vi "SW-Microscoper.vi"(1 "Number of Scans to Average":i32=1 min=1 max=10000 step=1, 2 "Integration Time (ms)":i32=20 caption="Inter scan delay ms" min=10 step=10) -> ()   [LabVIEW 2012]
uses:
  Spectrometer/Events/SpectrometerEvents.ctl
  typedefs/Filenaming.ctl
  Spectrometer/SpectrometerSpectraWiz.llb/StellarNet Globals.vi
  variables/GlobalUI.vi
  <vilib>/Utility/file.llb/Write To Spreadsheet File (string).vi
  <vilib>/Utility/file.llb/Write To Spreadsheet File (DBL).vi
panel:
  in  "1000 ms":bool
  in  "20ms":bool
  in  "File Description":string
  out "Intensity":dbl
  out "Wavelength":dbl
  in  "Watts":bool=TRUE
  in  "Normalize":bool
  in  "Enable fit":bool
  in  "Reset Graph":bool
  out "FWHM":dbl=12.0
  out "Center (nm)":dbl=785.070003461609
  in  "Offset":dbl step=500.0
  in  "FWHM":dbl=12.0
  out "Background":sgl[][](array[numeric])
  in  "Continuous":bool
  out "Spectrometer data array sizes":i32[](array[numeric])=[2047]
  out "Spectrometer wavelengths":sgl[][](array[numeric])=[[337.41, 337.9242, 338.4383, 338.95227, 339.46616, 339.97992, 340.4936, 341.00717, 341.52063, 342.03397, 342.54724, 343.06036, 343.57343, 344.08633, 344.59918, 345.11188, 345.6245, 346.13702, 346.6494, 347.1617, 347.67392, 348.186, 348.698, 349.20987, 349.72165, 350.2333, 350.74487, 351.25632, 351.76767, 352.27893, 352.79007, 353.30112, 353.81204, 354.32285, 354.8336, 355.34418, 355.8547, 356.3651, 356.8754, 357.3856, 357.8957, 358.40567, 358.91553, 359.4253, 359.93497, 360.44452, 360.95398, 361.46335, 361.97256, 362.48172, 362.99075, 363.49966, 364.0085, 364.5172, 365.02582, 365.53433, 366.04272, 366.55103, 367.0592, 367.5673, 368.0753, 368.58316, 369.0909, 369.59857, 370.10614, 370.6136, 371.12094, 371.62817, 372.1353, 372.64233, 373.14926, 373.6561, 374.1628, 374.6694, 375.1759, 375.6823, 376.1886, 376.6948, 377.20087, 377.70685, 378.2127, 378.71848, 379.22415, 379.7297, 380.23514, 380.74048, 381.24573, 381.75085, 382.2559, 382.7608, 383.26562, 383.77036, 384.27493, 384.77945, 385.28384, 385.78815, 386.29233, 386.7964, 387.30035, 387.80423, 388.308, 388.81165, 389.31522, 389.81866, 390.322, 390.82523, 391.32837, 391.8314, 392.33432, 392.83713, 393.33984, 393.84244, 394.34494, 394.84732, 395.3496, 395.8518, 396.35388, 396.85583, 397.3577, 397.85947, 398.3611, 398.86267, 399.3641, 399.86545, 400.3667, 400.8678, 401.36884, 401.86975, 402.37057, 402.87128, 403.37186, 403.87238, 404.37274, 404.87305, 405.37323, 405.8733, 406.37326, 406.87314, 407.3729, 407.87253, 408.37207, 408.87152, 409.37085, 409.8701, 410.3692, 410.86823, 411.36716, 411.86597, 412.36465, 412.86325, 413.36176, 413.86014, 414.35843, 414.8566, 415.35468, 415.85263, 416.3505, 416.84824, 417.3459, 417.84344, 418.34088, 418.83823, 419.33545, 419.83255, 420.3296, 420.8265, 421.3233, 421.82, 422.3166, 422.81308, 423.30948, 423.80576, 424.3019, 424.798, 425.29395, 425.78983, 426.28555, 426.78122, 427.27676, 427.7722, 428.26752, 428.76276, 429.25787, 429.75287, 430.2478, 430.74258, 431.2373, 431.73187, 432.22638, 432.72076, 433.21503, 433.7092, 434.20328, 434.69724, 435.19107, 435.68484, 436.17847, 436.67203, 437.16544, 437.65878, 438.152, 438.6451, 439.13812, 439.63104, 440.12384, 440.61655, 441.10913, 441.6016, 442.094, 442.58627, 443.07843, 443.5705, 444.06244, 444.5543, 445.04605, 445.5377, 446.02924, 446.52066, 447.012, 447.5032, 447.99432, 448.48532, 448.97623, 449.46704, 449.95773, 450.4483, 450.93878, 451.42917, 451.91943, 452.4096, 452.89966, 453.38962, 453.8795, 454.36923, 454.85886, 455.3484, 455.83783, 456.32715, 456.81638, 457.30548, 457.7945, 458.2834, 458.7722, 459.26086, 459.74945, 460.23795, 460.72632, 461.21457, 461.70273, 462.1908, 462.67874, 463.1666, 463.65433, 464.14197, 464.62952, 465.11694, 465.60425, 466.09146, 466.57858, 467.06558, 467.5525, 468.03928, 468.52597, 469.01254, 469.49902, 469.98538, 470.47165, 470.95782, 471.44388, 471.92984, 472.41568, 472.9014, 473.38705, 473.87256, 474.358, 474.84332, 475.32852, 475.81363, 476.29865, 476.78354, 477.2683, 477.753, 478.23758, 478.72205, 479.20642, 479.6907, 480.17487, 480.6589, 481.14285, 481.62668, 482.11044, 482.59406, 483.07758, 483.561, 484.0443, 484.52753, 485.01065, 485.49362, 485.97653, 486.45932, 486.942, 487.4246, 487.90704, 488.3894, 488.87167, 489.35382, 489.83588, 490.31784, 490.79965, 491.2814, 491.76303, 492.24457, 492.72598, 493.20728, 493.68848, 494.1696, 494.65057, 495.13147, 495.61227, 496.09296, 496.57352, 497.054, 497.53436, 498.01462, 498.49475, 498.97482, 499.45474, 499.9346, 500.41434, 500.89395, 501.37347, 501.85287, 502.33218, 502.8114, 503.2905, 503.7695, 504.24838, 504.72717, 505.20584, 505.68442, 506.16287, 506.64124, 507.1195, 507.59766, 508.07568, 508.55362, 509.03146, 509.5092, 509.98682, 510.46432, 510.94174, 511.41907, 511.89627, 512.37335, 512.85034, 513.3272, 513.804, 514.2807, 514.75726, 515.2337, 515.7101, 516.18634, 516.6625, 517.13855, 517.61444, 518.0903, 518.56604, 519.0416, 519.51715, 519.99255, 520.4679, 520.94305, 521.41815, 521.8931, 522.36804, 522.84283, 523.3175, 523.79205, 524.26654, 524.74084, 525.21515, 525.6893, 526.1633, 526.63727, 527.1111, 527.5848, 528.0584, 528.5319, 529.0053, 529.47864, 529.95184, 530.4249, 530.8979, 531.3708, 531.84357, 532.3162, 532.7888, 533.2612, 533.7336, 534.2059, 534.678, 535.15, 535.62195, 536.0938, 536.5655, 537.0371, 537.50867, 537.98004, 538.45135, 538.92255, 539.3936, 539.8646, 540.3355, 540.8063, 541.2769, 541.7475, 542.21796, 542.6883, 543.15857, 543.62866, 544.0987, 544.56866, 545.03845, 545.5082, 545.9778, 546.4473, 546.9167, 547.386, 547.8552, 548.3243, 548.7933, 549.26215, 549.7309, 550.1996, 550.66815, 551.1366, 551.6049, 552.0732, 552.5413, 553.00934, 553.4773, 553.9451, 554.41284, 554.88043, 555.34796, 555.8153, 556.28265, 556.7498, 557.2169, 557.6839, 558.15076, 558.6175, 559.08417, 559.5507, 560.0172, 560.4835, 560.94977, 561.4159, 561.88196, 562.34784, 562.81366, 563.2794, 563.745, 564.2105, 564.6759, 565.1412, 565.6064, 566.0715, 566.53644, 567.0013, 567.46606, 567.9307, 568.39526, 568.85974, 569.3241, 569.7883, 570.25244, 570.7165, 571.1804, 571.6442, 572.1079, 572.57153, 573.03503, 573.4984, 573.96173, 574.42487, 574.888, 575.35095, 575.8138, 576.27655, 576.73926, 577.2018, 577.66425, 578.1266, 578.5888, 579.0509, 579.51294, 579.97485, 580.4367, 580.8984, 581.36, 581.8215, 582.2829, 582.7442, 583.2054, 583.66644, 584.1274, 584.58826, 585.049, 585.5097, 585.9702, 586.43066, 586.891, 587.35126, 587.81134, 588.27136, 588.7313, 589.1911, 589.6508, 590.1104, 590.56995, 591.0293, 591.4886, 591.94775, 592.40686, 592.8658, 593.32465, 593.78345, 594.24207, 594.7006, 595.15906, 595.61743, 596.0756, 596.53375, 596.99176, 597.4497, 597.9075, 598.3652, 598.8228, 599.2803, 599.7377, 600.19495, 600.65216, 601.1092, 601.56616, 602.023, 602.4798, 602.93646, 603.393, 603.8494, 604.3057, 604.76196, 605.2181, 605.67413, 606.13, 606.5858, 607.0415, 607.49713, 607.95264, 608.408, 608.8633, 609.3185, 609.7735, 610.22845, 610.68335, 611.1381, 611.5927, 612.0473, 612.5017, 612.95605, 613.4103, 613.8644, 614.3184, 614.77234, 615.22614, 615.6798, 616.1334, 616.5869, 617.0403, 617.4935, 617.9467, 618.3998, 618.8527, 619.3056, 619.75836, 620.211, 620.6635, 621.11597, 621.5683, 622.0205, 622.47266, 622.9246, 623.3765, 623.82837, 624.28, 624.7316, 625.1831, 625.6345, 626.08575, 626.5369, 626.988, 627.43896, 627.88983, 628.3406, 628.7912, 629.24176, 629.69214, 630.1425, 630.5927, 631.04285, 631.49286, 631.94275, 632.3925, 632.8422, 633.2918, 633.7413, 634.1907, 634.63995, 635.0891, 635.53815, 635.9871, 636.436, 636.8847, 637.3334, 637.78186, 638.2303, 638.67865, 639.12683, 639.57495, 640.02295, 640.4709, 640.91864, 641.36633, 641.81396, 642.2614, 642.7088, 643.15607, 643.6032, 644.0503, 644.49725, 644.9441, 645.3908, 645.83746, 646.284, 646.7304, 647.17676, 647.6229, 648.06903, 648.5151, 648.96094, 649.40674, 649.8524, 650.29803, 650.74347, 651.18884, 651.63416, 652.0793, 652.52435, 652.9693, 653.4141, 653.8589, 654.3035, 654.74805, 655.19244, 655.6368, 656.081, 656.5251, 656.9691, 657.413, 657.8568, 658.3005, 658.7441, 659.1875, 659.6309, 660.07416, 660.51733, 660.9604, 661.4033, 661.8461, 662.2889, 662.7315, 663.1741, 663.61646, 664.0588, 664.501, 664.9431, 665.3851, 665.82697, 666.2688, 666.71045, 667.15204, 667.5935, 668.03485, 668.47614, 668.9173, 669.35834, 669.79926, 670.2401, 670.68085, 671.12146, 671.562, 672.00244, 672.44275, 672.88293, 673.32306, 673.76306, 674.20294, 674.6427, 675.0824, 675.522, 675.9614, 676.4008, 676.84, 677.2792, 677.71826, 678.15717, 678.596, 679.0348, 679.4734, 679.9119, 680.35034, 680.78864, 681.2268, 681.6649, 682.1029, 682.54083, 682.9786, 683.41626, 683.8538, 684.2913, 684.7287, 685.16595, 685.6031, 686.0401, 686.47705, 686.9139, 687.35065, 687.78723, 688.22375, 688.66016, 689.0965, 689.53265, 689.96875, 690.4048, 690.84064, 691.2764, 691.7121, 692.1477, 692.5831, 693.0185, 693.45374, 693.8889, 694.3239, 694.75885, 695.1937, 695.6284, 696.06305, 696.49756, 696.932, 697.3663, 697.8005, 698.23456, 698.6686, 699.1024, 699.5362, 699.9699, 700.40344, 700.8369, 701.27026, 701.70355, 702.13666, 702.5697, 703.0026, 703.4355, 703.8682, 704.30084, 704.73334, 705.1657, 705.598, 706.0302, 706.46234, 706.8943, 707.3262, 707.75793, 708.18964, 708.6212, 709.0527, 709.484, 709.9152, 710.3464, 710.7774, 711.2084, 711.63916, 712.0699, 712.50055, 712.931, 713.36145, 713.79175, 714.2219, 714.65204, 715.082, 715.5119, 715.94165, 716.37134, 716.8009, 717.23035, 717.65967, 718.0889, 718.51807, 718.9471, 719.37604, 719.8049, 720.2336, 720.6622, 721.0907, 721.5191, 721.9474, 722.37555, 722.80365, 723.2316, 723.65955, 724.0873, 724.51495, 724.9425, 725.37, 725.7973, 726.22455, 726.6517, 727.07874, 727.5057, 727.9325, 728.3592, 728.78577, 729.2123, 729.6387, 730.065, 730.4912, 730.91724, 731.34326, 731.7691, 732.1949, 732.62054, 733.0461, 733.47156, 733.8969, 734.32214, 734.74725, 735.1723, 735.5972, 736.02203, 736.4468, 736.87134, 737.29584, 737.7203, 738.14453, 738.5687, 738.9928, 739.4168, 739.84064, 740.2644, 740.6881, 741.11163, 741.5351, 741.95844, 742.38165, 742.8048, 743.22784, 743.65076, 744.07355, 744.4963, 744.9189, 745.3414, 745.76373, 746.18604, 746.6082, 747.03033, 747.4523, 747.87415, 748.2959, 748.7176, 749.1391, 749.56055, 749.98193, 750.40314, 750.8243, 751.2453, 751.6662, 752.08704, 752.50775, 752.92834, 753.3488, 753.7692, 754.1895, 754.6097, 755.0298, 755.4497, 755.86957, 756.28937, 756.709, 757.12854, 757.548, 757.96735, 758.3866, 758.8057, 759.22473, 759.6436, 760.06244, 760.48114, 760.8997, 761.31824, 761.73663, 762.1549, 762.5731, 762.99115, 763.4091, 763.82697, 764.24475, 764.6624, 765.07996, 765.4974, 765.91473, 766.332, 766.7491, 767.1661, 767.583, 767.9998, 768.4165, 768.8331, 769.2496, 769.666, 770.0823, 770.4985, 770.9145, 771.3305, 771.74634, 772.1621, 772.57776, 772.9933, 773.4087, 773.82404, 774.23926, 774.6544, 775.0694, 775.4843, 775.8991, 776.31384, 776.72845, 777.14294, 777.5573, 777.97156, 778.38574, 778.7998, 779.2138, 779.6276, 780.0414, 780.455, 780.8686, 781.282, 781.6953, 782.1086, 782.52167, 782.9347, 783.3476, 783.7604, 784.1731, 784.5857, 784.99817, 785.4106, 785.8228, 786.235, 786.6471, 787.059, 787.4709, 787.8826, 788.29425, 788.7058, 789.11725, 789.52856, 789.9398, 790.3509, 790.7619, 791.17285, 791.5836, 791.9943, 792.4049, 792.81537, 793.22577, 793.63605, 794.0462, 794.4563, 794.8662, 795.27606, 795.68585, 796.09546, 796.505, 796.9144, 797.3237, 797.733, 798.1421, 798.5511, 798.96, 799.3688, 799.77747, 800.1861, 800.59454, 801.0029, 801.4112, 801.8194, 802.2274, 802.6354, 803.0432, 803.451, 803.8586, 804.2661, 804.6736, 805.0809, 805.4881, 805.8952, 806.30225, 806.7091, 807.1159, 807.5226, 807.9292, 808.3357, 808.74207, 809.1483, 809.5545, 809.9605, 810.36646, 810.77234, 811.17804, 811.5837, 811.98926, 812.39465, 812.8, 813.2052, 813.6103, 814.0153, 814.4202, 814.825, 815.2297, 815.6343, 816.03876, 816.4431, 816.84735, 817.2515, 817.6556, 818.0595, 818.4634, 818.8671, 819.27075, 819.67426, 820.0777, 820.481, 820.8842, 821.28735, 821.6903, 822.0932, 822.49603, 822.8987, 823.3013, 823.70374, 824.10614, 824.50836, 824.9105, 825.3126, 825.71454, 826.1164, 826.5181, 826.91974, 827.3213, 827.7227, 828.124, 828.5252, 828.92633, 829.32733, 829.7282, 830.12897, 830.52966, 830.93024, 831.33075, 831.7311, 832.13135, 832.5315, 832.9315, 833.3315, 833.7313, 834.13104, 834.5307, 834.93024, 835.32965, 835.72894, 836.1282, 836.5272, 836.9263, 837.32513, 837.72394, 838.1226, 838.5212, 838.9196, 839.318, 839.71625, 840.1144, 840.51245, 840.9104, 841.3082, 841.70593, 842.1036, 842.5011, 842.8985, 843.29584, 843.69305, 844.09015, 844.4871, 844.88403, 845.2808, 845.6775, 846.07404, 846.4705, 846.8669, 847.2631, 847.65924, 848.0553, 848.45123, 848.8471, 849.2428, 849.6384, 850.03394, 850.4294, 850.82465, 851.21985, 851.615, 852.00995, 852.40485, 852.7996, 853.1943, 853.58887, 853.98334, 854.3777, 854.7719, 855.1661, 855.5601, 855.95404, 856.3479, 856.74164, 857.13525, 857.52875, 857.9222, 858.3154, 858.7087, 859.10175, 859.49475, 859.88763, 860.2804, 860.6731, 861.0656, 861.45807, 861.85046, 862.2427, 862.6348, 863.02686, 863.4188, 863.81067, 864.2024, 864.594, 864.9855, 865.3769, 865.7682, 866.1594, 866.5505, 866.94147, 867.33234, 867.72314, 868.1138, 868.50433, 868.89484, 869.28516, 869.6754, 870.06555, 870.45557, 870.8455, 871.23535, 871.62506, 872.0147, 872.4042, 872.7936, 873.18286, 873.5721, 873.9612, 874.35016, 874.739, 875.1278, 875.5165, 875.905, 876.29346, 876.6818, 877.07007, 877.4582, 877.84625, 878.2342, 878.622, 879.0097, 879.39734, 879.78485, 880.17224, 880.5595, 880.9467, 881.3338, 881.72076, 882.10767, 882.49445, 882.8811, 883.26764, 883.6541, 884.04047, 884.4267, 884.8128, 885.19885, 885.5848, 885.9706, 886.3563, 886.74194, 887.12744, 887.5128, 887.89813, 888.2833, 888.6684, 889.05334, 889.43823, 889.823, 890.20764, 890.5922, 890.9767, 891.361, 891.74524, 892.1294, 892.5134, 892.89734, 893.2812, 893.66486, 894.04846, 894.432, 894.81537, 895.19867, 895.58185, 895.9649, 896.3479, 896.7308, 897.1135, 897.4962, 897.8787, 898.26117, 898.64355, 899.02576, 899.4079, 899.7899, 900.1719, 900.55365, 900.93536, 901.31696, 901.6985, 902.0799, 902.4612, 902.84235, 903.22345, 903.6044, 903.9852, 904.366, 904.7467, 905.1272, 905.5077, 905.888, 906.26825, 906.6484, 907.0284, 907.4083, 907.78815, 908.16785, 908.5474, 908.92694, 909.30634, 909.6856, 910.06476, 910.44385, 910.8228, 911.2017, 911.58044, 911.9591, 912.33765, 912.71606, 913.0944, 913.47266, 913.85077, 914.2288, 914.60675, 914.98456, 915.36224, 915.7398, 916.1173, 916.4947, 916.872, 917.2492, 917.6262, 918.00323, 918.38007, 918.75684, 919.1335, 919.51, 919.8865, 920.2628, 920.63904, 921.01514, 921.3912, 921.7671, 922.1429, 922.5186, 922.89417, 923.26965, 923.6451, 924.0203, 924.3955, 924.77057, 925.14557, 925.5204, 925.89514, 926.26984, 926.64435, 927.0188, 927.3931, 927.76733, 928.1415, 928.5155, 928.8894, 929.2632, 929.6369, 930.0105, 930.384, 930.7574, 931.1306, 931.5038, 931.8769, 932.2498, 932.6227, 932.9954, 933.3681, 933.74066, 934.11304, 934.4854, 934.8576, 935.22974, 935.60175, 935.97363, 936.34546, 936.71716, 937.08875, 937.4602, 937.8316, 938.2029, 938.57404, 938.9451, 939.3161, 939.68695, 940.0577, 940.42834, 940.7989, 941.1693, 941.5396, 941.90985, 942.27997, 942.64996, 943.0199, 943.38965, 943.75934, 944.12897, 944.4984, 944.8678, 945.23706, 945.60626, 945.97534, 946.3443, 946.71313, 947.08185, 947.4505, 947.81903, 948.18744, 948.5558, 948.924, 949.2921, 949.66016, 950.028, 950.3958, 950.76355, 951.1311, 951.4986, 951.86597, 952.2332, 952.6004, 952.96747, 953.3344, 953.70123, 954.068, 954.43463, 954.80115, 955.1676, 955.53394, 955.90015, 956.26624, 956.63226, 956.99817, 957.36395, 957.7296, 958.0952, 958.4607, 958.82605, 959.19135, 959.5565, 959.9216, 960.2865, 960.65137, 961.0161, 961.38074, 961.74524, 962.1097, 962.474, 962.8382, 963.20233, 963.56635, 963.93024, 964.294, 964.6577, 965.02124, 965.38477, 965.7481, 966.1114, 966.47455, 966.8376, 967.20056, 967.56335, 967.92615, 968.28876, 968.6513, 969.0137, 969.37604, 969.7382, 970.10034, 970.46234, 970.8242, 971.18604, 971.5477, 971.9093, 972.27075, 972.63214, 972.9934, 973.35455, 973.7156, 974.07654, 974.4374, 974.7981, 975.15875, 975.5193, 975.8797, 976.24, 976.6002, 976.9603, 977.3203, 977.6802, 978.04, 978.39966, 978.7592, 979.1187, 979.4781, 979.83734, 980.1965, 980.55554, 980.9145, 981.2733, 981.632, 981.99066, 982.3492, 982.7076, 983.0659, 983.42413, 983.7822, 984.1402, 984.4981, 984.8559, 985.21356, 985.57117, 985.9286, 986.28595, 986.64325, 987.00037, 987.3574, 987.71436, 988.0712, 988.4279, 988.78455, 989.14105, 989.4975, 989.8538, 990.21, 990.5661, 990.9221, 991.27795, 991.6337, 991.98944, 992.34503, 992.70044, 993.05585, 993.4111, 993.76624, 994.1213, 994.4762, 994.83105, 995.1858, 995.5404, 995.8949, 996.2493, 996.60364, 996.9578, 997.3119, 997.6659, 998.0198, 998.3736, 998.72723, 999.0808, 999.43427, 999.78766, 1000.14087, 1000.494, 1000.84705, 1001.2, 1001.55286, 1001.9056, 1002.2582, 1002.6107, 1002.9631, 1003.3154, 1003.6676, 1004.0197, 1004.3717, 1004.7236, 1005.0753, 1005.427, 1005.77856, 1006.13, 1006.4814, 1006.83264, 1007.1838, 1007.5348, 1007.88574, 1008.2366, 1008.5873, 1008.9379, 1009.28845, 1009.63885, 1009.98914, 1010.33936, 1010.6894, 1011.0394, 1011.3893, 1011.7391, 1012.08875, 1012.4383, 1012.7877, 1013.1371, 1013.4863, 1013.83545, 1014.1845, 1014.53345, 1014.88226, 1015.231, 1015.5796, 1015.9281, 1016.2765, 1016.6248, 1016.973, 1017.3211, 1017.66907, 1018.01697, 1018.36475, 1018.7124, 1019.05994, 1019.4074, 1019.75476, 1020.102, 1020.44916, 1020.79614, 1021.14307, 1021.4899, 1021.8366, 1022.1832, 1022.5297, 1022.87616, 1023.2225, 1023.5686, 1023.91473, 1024.2607, 1024.6066, 1024.9524, 1025.298, 1025.6436, 1025.989, 1026.3344, 1026.6796, 1027.0248, 1027.3698, 1027.7147, 1028.0594, 1028.4042, 1028.7488, 1029.0934, 1029.4377, 1029.782, 1030.1262, 1030.4703, 1030.8142, 1031.1581, 1031.502, 1031.8456, 1032.1891, 1032.5326, 1032.8759, 1033.2191, 1033.5623, 1033.9053, 1034.2483, 1034.5911, 1034.9337, 1035.2764, 1035.6189, 1035.9613, 1036.3036, 1036.6458, 1036.9878, 1037.3298, 1037.6716, 1038.0134, 1038.3551, 1038.6967, 1039.0381, 1039.3794, 1039.7207, 1040.0618, 1040.4028, 1040.7438, 1041.0846, 1041.4253, 1041.7659, 1042.1063, 1042.4468, 1042.787, 1043.1272, 1043.4673, 1043.8073, 1044.1471, 1044.4869, 1044.8265, 1045.1661, 1045.5055, 1045.8448, 1046.1841, 1046.5232, 1046.8623, 1047.2012, 1047.54, 1047.8787, 1048.2173, 1048.5558, 1048.8942, 1049.2324, 1049.5707, 1049.9087, 1050.2467, 1050.5846, 1050.9224, 1051.26, 1051.5975, 1051.9349, 1052.2723, 1052.6095, 1052.9467, 1053.2837, 1053.6206, 1053.9574, 1054.2941, 1054.6307, 1054.9672, 1055.3036, 1055.6399, 1055.9761, 1056.3121, 1056.6481, 1056.9839, 1057.3197, 1057.6553, 1057.9908, 1058.3263, 1058.6616, 1058.9968, 1059.332, 1059.667, 1060.002, 1060.3368, 1060.6714, 1061.006, 1061.3406, 1061.6749, 1062.0092, 1062.3434, 1062.6775, 1063.0114, 1063.3452, 1063.679, 1064.0127, 1064.3462, 1064.6797, 1065.013, 1065.3462, 1065.6793, 1066.0123, 1066.3452, 1066.678, 1067.0107, 1067.3434, 1067.6758, 1068.0082, 1068.3405, 1068.6726, 1069.0048, 1069.3367, 1069.6686, 1070.0002, 1070.3319, 1070.6635, 1070.9949, 1071.3262, 1071.6575, 1071.9885, 1072.3196, 1072.6505, 1072.9813, 1073.312, 1073.6426, 1073.973, 1074.3035, 1074.6337, 1074.9639, 1075.294, 1075.6239, 1075.9537, 1076.2834, 1076.6132, 1076.9426, 1077.2721, 1077.6014, 1077.9307, 1078.2598, 1078.5887, 1078.9177, 1079.2465, 1079.5752, 1079.9038, 1080.2323, 1080.5607, 1080.8889, 1081.217, 1081.5452, 1081.873, 1082.2009, 1082.5287, 1082.8563, 1083.1838, 1083.5112, 1083.8386, 1084.1658, 1084.4929, 1084.82, 1085.1469, 1085.4736, 1085.8003, 1086.127, 1086.4534, 1086.7798, 1087.1061, 1087.4323, 1087.7583, 1088.0842, 1088.41, 1088.7358, 1089.0614, 1089.387, 1089.7124, 1090.0377, 1090.3629, 1090.688, 1091.0131, 1091.3379, 1091.6627, 1091.9874, 1092.312, 1092.6365, 1092.9608, 1093.2852, 1093.6093, 1093.9333, 1094.2573, 1094.5812, 1094.9049, 1095.2285, 1095.552, 1095.8755, 1096.1987, 1096.522, 1096.8451, 1097.1681, 1097.491, 1097.8137, 1098.1365, 1098.459, 1098.7815, 1099.1039, 1099.4261, 1099.7483, 1100.0703, 1100.3923, 1100.7141, 1101.0359, 1101.3575, 1101.6791, 1102.0005, 1102.3218, 1102.643, 1102.9641, 1103.2852, 1103.606, 1103.9268, 1104.2474, 1104.568, 1104.8885, 1105.2089, 1105.5292, 1105.8492, 1106.1693, 1106.4893, 1106.8091, 1107.1289, 1107.4485, 1107.7681, 1108.0874, 1108.4067, 1108.726, 1109.045, 1109.364, 1109.683, 1110.0017, 1110.3204, 1110.639, 1110.9574, 1111.2759, 1111.5941, 1111.9122, 1112.2302, 1112.5482, 1112.8661, 1113.1838, 1113.5015, 1113.819, 1114.1364, 1114.4536, 1114.7709, 1115.088, 1115.4049, 1115.7218, 1116.0386, 1116.3553, 1116.6719, 1116.9884, 1117.3047, 1117.621, 1117.9371, 1118.2532, 1118.5691, 1118.8849, 1119.2007, 1119.5162, 1119.8318, 1120.1472, 1120.4625, 1120.7777, 1121.0928, 1121.4078, 1121.7227, 1122.0375, 1122.3522, 1122.6667, 1122.9812, 1123.2955, 1123.6099, 1123.924, 1124.238, 1124.5519, 1124.8657, 1125.1794, 1125.4932, 1125.8066, 1126.12, 1126.4333, 1126.7466, 1127.0597, 1127.3727, 1127.6855, 1127.9983, 1128.3109, 1128.6235, 1128.936, 1129.2483, 1129.5605, 1129.8728, 1130.1848, 1130.4967, 1130.8086, 1131.1202, 1131.4319, 1131.7434, 1132.0548, 1132.3661, 1132.6774, 1132.9884, 1133.2994, 1133.6102, 1133.921, 1134.2317, 1134.5422, 1134.8528, 1135.1631, 1135.4734, 1135.7834, 1136.0935, 1136.4034, 1136.7133, 1137.023, 1137.3326, 1137.6421, 1137.9515, 1138.2609, 1138.5701, 1138.8792, 1139.1881, 1139.497, 1139.8058, 1140.1144, 1140.423, 1140.7314, 1141.0398, 1141.348, 1141.6561, 1141.9642, 1142.2721, 1142.58, 1142.8877, 1143.1953, 1143.5028, 1143.8102, 1144.1176, 1144.4247, 1144.7318, 1145.0388, 1145.3456, 1145.6525, 1145.9591, 1146.2656, 1146.5721, 1146.8784, 1147.1847, 1147.4908, 1147.7969, 1148.1028, 1148.4086, 1148.7144, 1149.0199, 1149.3254, 1149.6309, 1149.9362, 1150.2413, 1150.5464, 1150.8513, 1151.1562, 1151.461, 1151.7656, 1152.0702, 1152.3746, 1152.6791, 1152.9833, 1153.2874, 1153.5914, 1153.8954, 1154.1992, 1154.5029, 1154.8065, 1155.11, 1155.4135, 1155.7167, 1156.0199, 1156.323, 1156.626, 1156.9288, 1157.2316, 1157.5342, 1157.8368, 1158.1393, 1158.4415, 1158.7438, 1159.0459, 1159.348, 1159.6499, 1159.9517, 1160.2534, 1160.555, 1160.8566, 1161.158, 1161.4592, 1161.7604, 1162.0615, 1162.3624, 1162.6633, 1162.9641, 1163.2648, 1163.5653, 1163.8657, 1164.166, 1164.4663, 1164.7665, 1165.0664, 1165.3663, 1165.6661, 1165.966, 1166.2655, 1166.565, 1166.8644, 1167.1637, 1167.4629, 1167.762, 1168.0609, 1168.3597, 1168.6586, 1168.9572]]
  out "time elapsed prev scan (ms)":u32=270
  in  "Acquire Background":bool
  in  "Array":bool[](array[boolean])=[TRUE, TRUE, TRUE]
  out "Save paths":path[](array[path])=[path "C:/Users/Trent/Documents/Jeremy/2016-09-27/FW800 with Polarizer-100mW-417mW-0mV-0mV-0mV-4xch1_s_00.csv", path "C:/Users/Trent/Documents/Jeremy/2016-09-27/FW800 with Polarizer-100mW-417mW-0mV-0mV-0mV-4xch2_s_00.csv", path "C:/Users/Trent/Documents/Jeremy/2016-09-27/FW800 with Polarizer-100mW-417mW-0mV-0mV-0mV-4xch3_s_00.csv"]
  out "Numeric":i32=623
  in  "Init Trigger":bool
  in  "Autosave":bool
  in  "Acquire Trigger":bool
  in  "STOP":bool
  out "Spectral history":cluster{sgl, "lamda":sgl}[](graph)=[{0.12466025, "lamda"=796.9144}, {0.0966606, "lamda"=681.83813}, {0.06927186, "lamda"=985.23456}]
  out "Spectrum":T1(graph)
  # "BlackComet"
  # "BlueWave"
  # "DwarfStar"
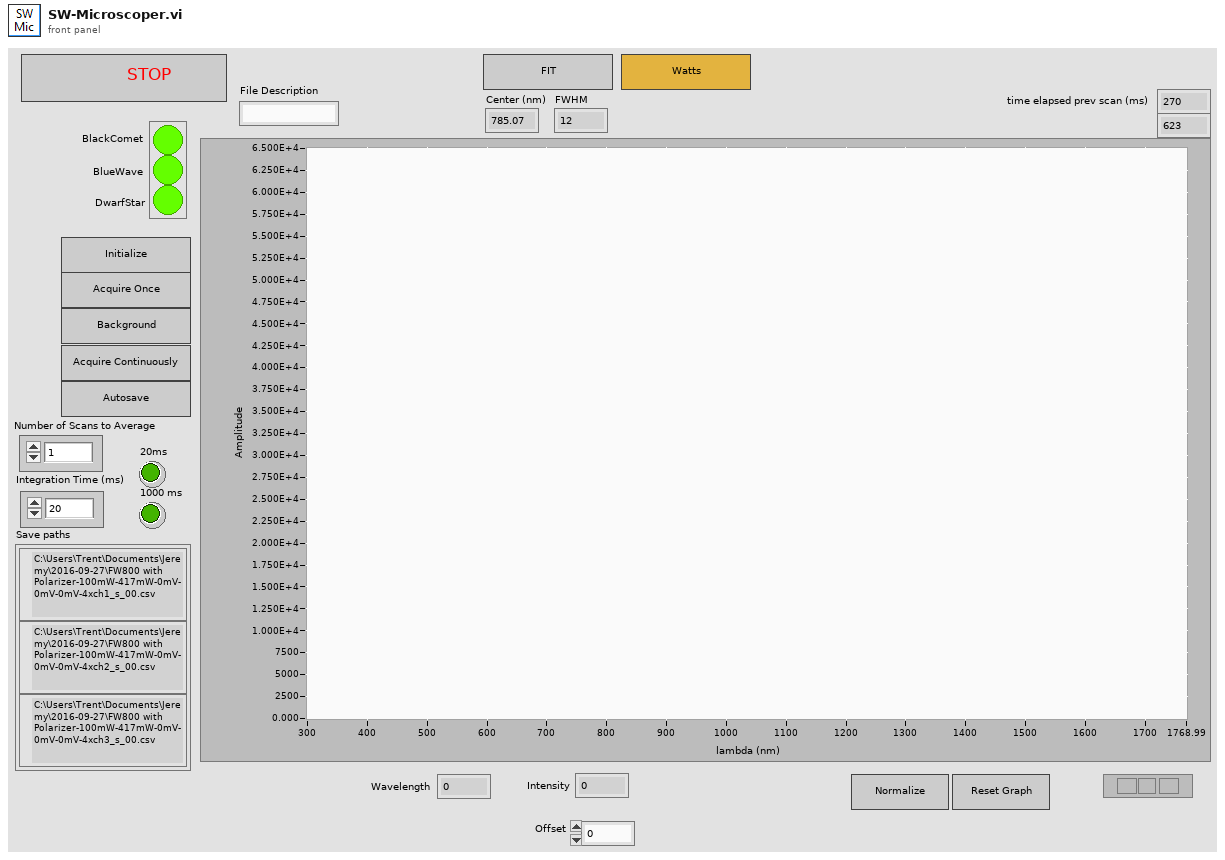
[diagram p1: front panel]
types:
  T1 = cluster{"Spectrometer wavelengths":sgl[], "buffer out":sgl[]}[]
  T2 = typedef "SpectrometerEvents.ctl" = enum16{"TimeOut", "Init Programmatically", "Init Button", "Init Background", "Acquire Background", "Acquire"}
  T3 = typedef "Filenaming.ctl" = enum16{"Image", "Just Description"}
  T4 = cluster{"Integration Time (msec)":i32, "Xtrate":i32, "Averaging":i32, "Smoothing":i32, "C1":dbl, "C2":dbl, "C3":dbl, "C4":dbl, "Digitizer Bits":enum8{"12", "14", "16"}}[]
  T5 = cluster{"Spectrometer wavelengths (filtered)":sgl[], "Normalized":dbl[]}
  T6 = cluster{"Spectrometer wavelengths (filtered)":sgl[], "Best Gaussian Fit":dbl[]}[]
  T7 = cluster{"Spectrometer wavelengths (filtered)":sgl[], "Normalized":sgl[]}
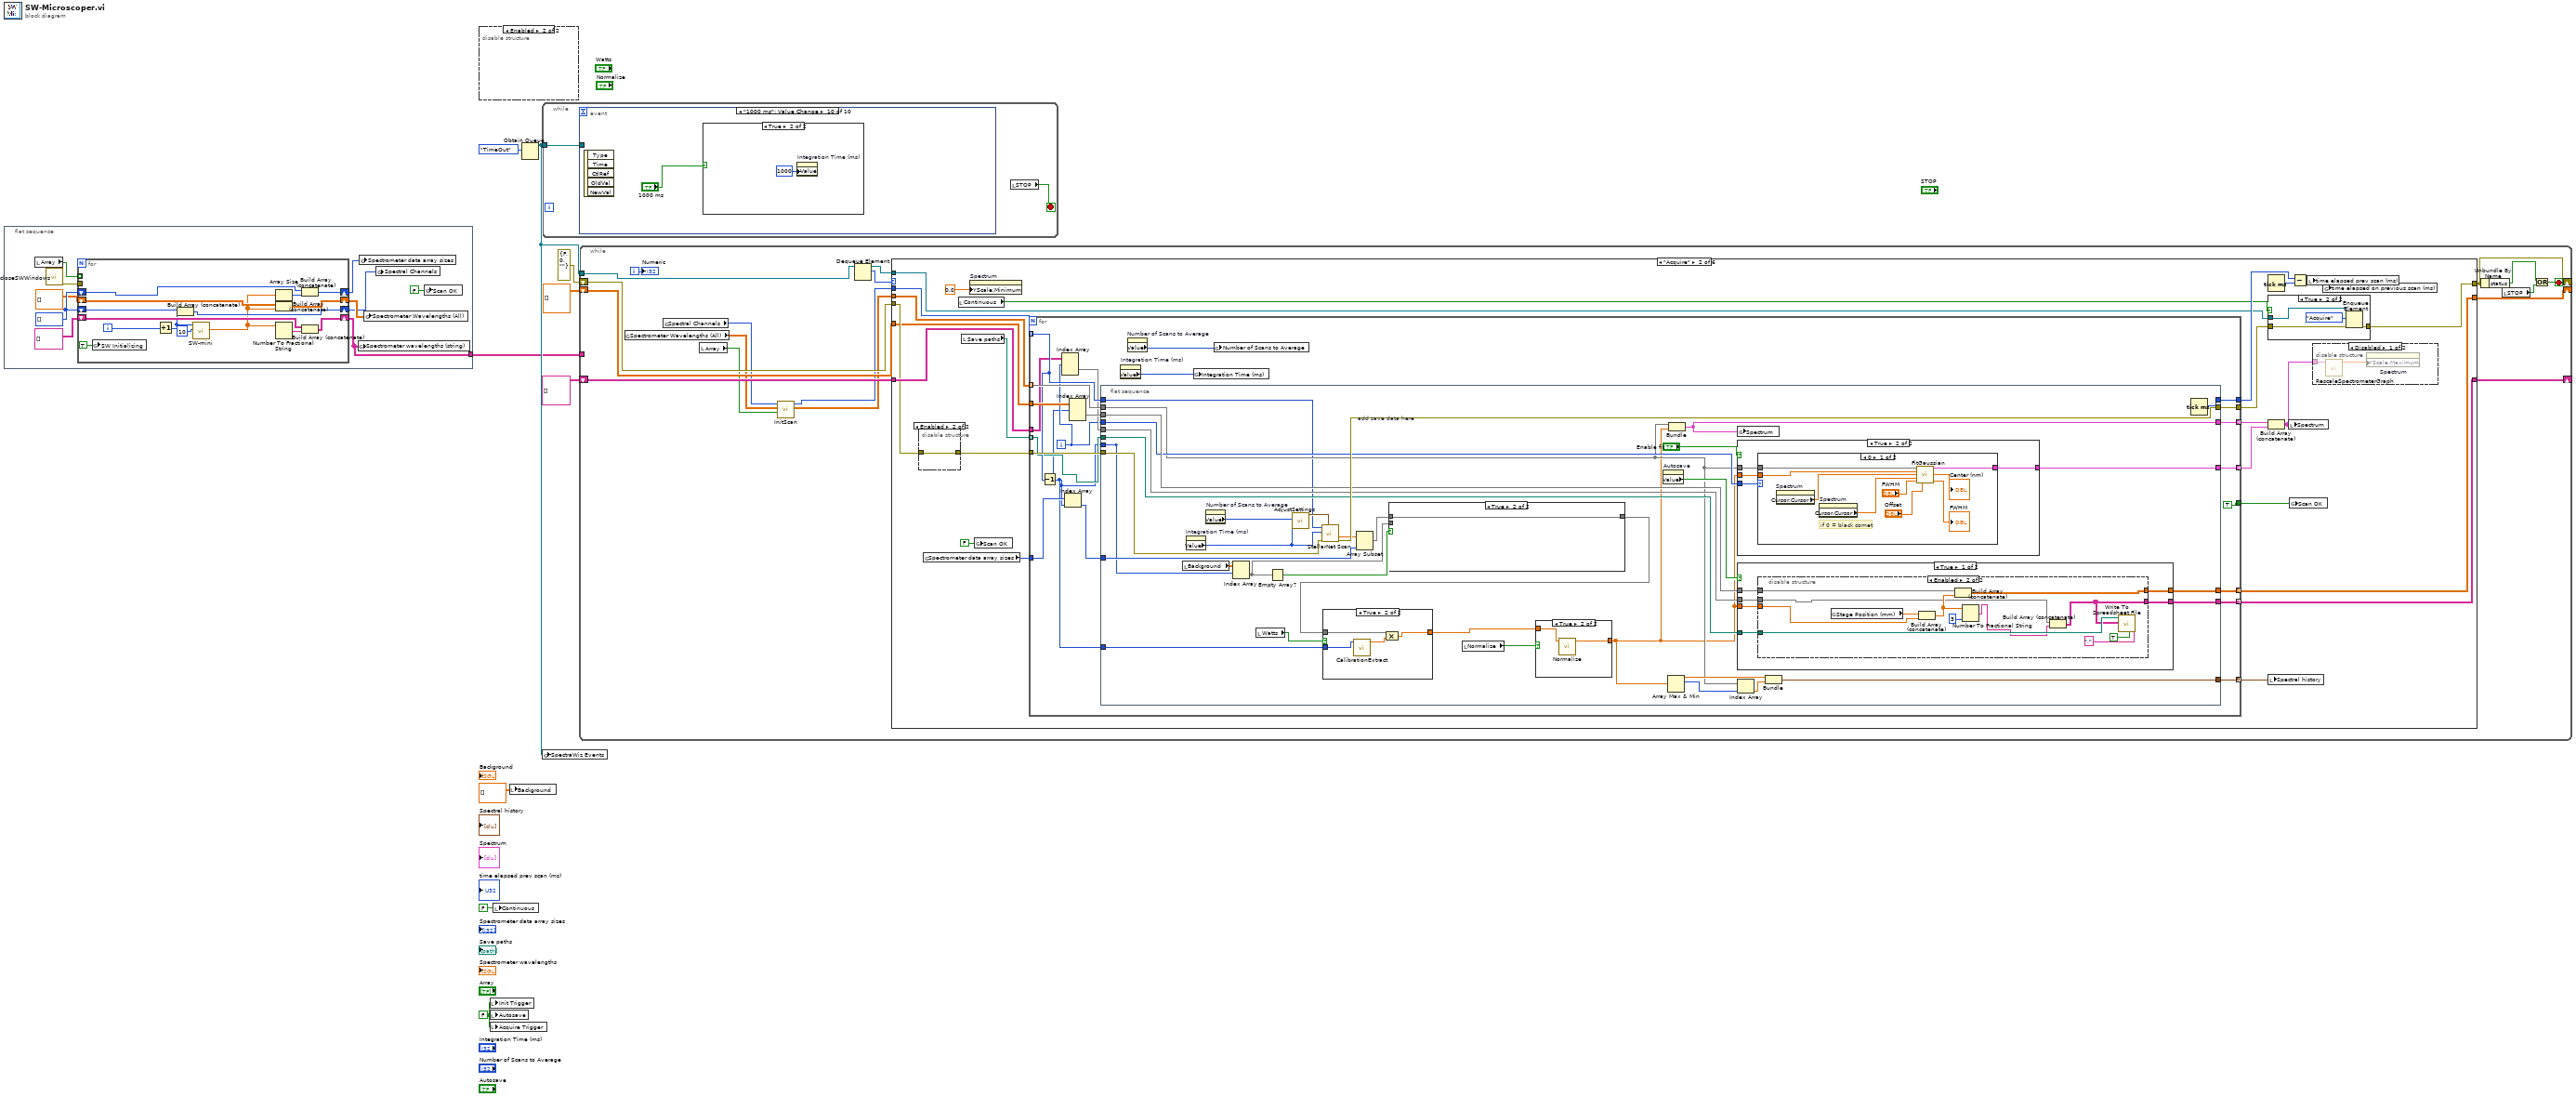
[diagram p0: block diagram]
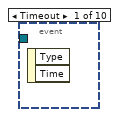
[diagram p2: hidden frame]
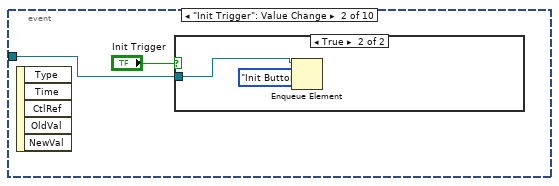
[diagram p3: hidden frame]
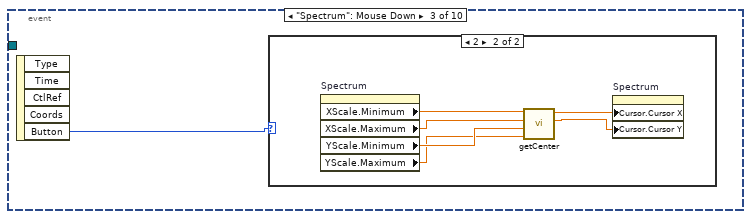
[diagram p5: hidden frame]
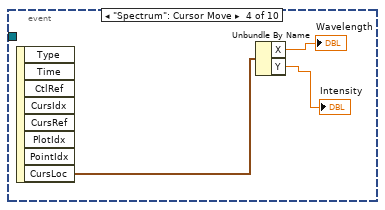
[diagram p7: hidden frame]
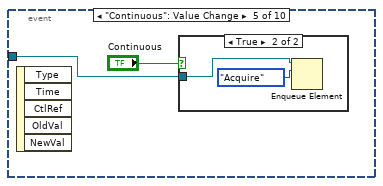
[diagram p8: hidden frame]
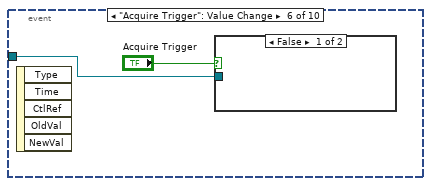
[diagram p10: hidden frame]
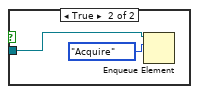
[diagram p11: hidden frame]
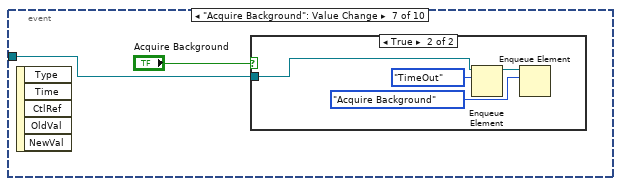
[diagram p12: hidden frame]
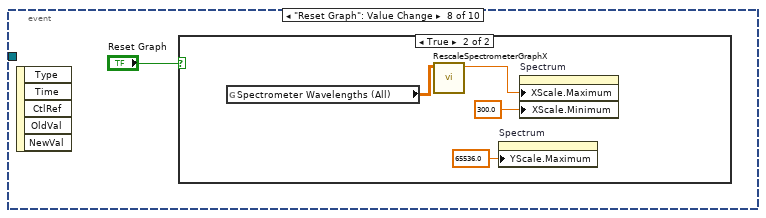
[diagram p14: hidden frame]
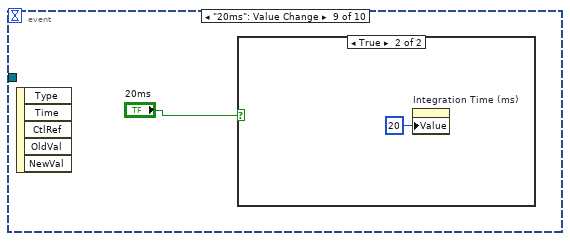
[diagram p16: hidden frame]
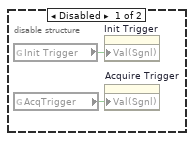
[diagram p19: hidden frame]
diagram:
  w2 = FALSE ("Init Trigger")
  n1 = flat-sequence {
    tunnel: [w11] -> w1
    frame #0 {
      w19 = i32[] []
      n2 = local read "Array"() -> (w17:bool[])
      n3 = call "closeSWWindows.vi"() -> ("error out"=w15:errorcluster)  [unwired: 11 in]
      n4 = for {
        tunnel: w17 -> [_] mode=indexing
        shift-right: [w33] -> w13
        shift-left: w19 -> [w32]
        tunnel: w15 -> [_]
        shift-right: [w30] -> w11
        shift-left: string[][] [] -> [w31]
        shift-right: [w28] -> w14
        shift-left: dbl[][] [] -> [w29]
        shift-right: [w27] -> w12
        shift-left: w19 -> [w26]
        i -> [w34]
        n5 = global write "GlobalUI.vi" "SW Initializing"(TRUE ("SW Initializing")) -> ()
        n6 = Increment(x=w34) -> (x+1=w25:i32)
        n7 = Build Array (concatenate)(w32, w25) -> (w33:i32[])
        n8 = call "SW-mini.vi"("Integration Time (ms)"=10, "Spectral Channel"=w25) -> ("Spectrometer wavelengths"=w22:sgl[])  [unwired: 6 in, 3 out]
        n9 = Array Size(array=w22) -> (size(s)=w21:i32)
        n10 = Build Array (concatenate)(w29, w22) -> (w28:dbl[][])
        n11 = Number To Fractional String(number=w22) -> (F-format string=w23:string[])  [unwired: 3 in]
        n12 = Build Array (concatenate)(w26, w21) -> (w27:i32[])
        n13 = Build Array (concatenate)(w31, w23) -> (w30:string[][])
      }
      n14 = global write "StellarNet Globals.vi" "Spectrometer wavelengths (string)"(w11) -> ()
      n15 = global write "StellarNet Globals.vi" "Spectrometer data array sizes"(w12) -> ()
      n16 = global write "StellarNet Globals.vi" "Spectrometer Wavelengths (All)"(w14) -> ()
      n17 = global write "StellarNet Globals.vi" "Spectral Channels"(w13) -> ()
      n18 = global write "StellarNet Globals.vi" "Scan OK"(FALSE ("Scan OK")) -> ()
    }
  }
  n19 = disable-structure shown="Enabled" {
    frame Disabled {
      n20 = global read "StellarNet Globals.vi" "Init Trigger"() -> (w36:bool)
      n21 = global read "StellarNet Globals.vi" "AcqTrigger"() -> (w35:bool)
      n22 = property on="Init Trigger" class="Bool (strict)"("Val(Sgnl)"=w36) -> ()  [unwired: 2 in, 2 out]
      n23 = property on="Acquire Trigger" class="Bool (strict)"("Val(Sgnl)"=w35) -> ()  [unwired: 2 in, 2 out]
    }
    frame Enabled {
    }
  }
  n24 = local write "Init Trigger"(w2) -> ()
  n25 = local write "Autosave"(w2) -> ()
  n26 = local write "Acquire Trigger"(w2) -> ()
  n27 = local write "Continuous"(FALSE ("Continuous")) -> ()
  n28 = local write "Background"(dbl[][] []) -> ()
  n29 = Obtain Queue(element data type=SpectrometerEvents."TimeOut" ("element")) -> (queue out=w5:refnum<queue>)  [unwired: 4 in, 2 out]
  n30 = while {
    tunnel: w5 -> [w38]
    stop <- w37 stop-if-true
    n31 = event shown="[9] \"1000 ms\": Value Change" {
      selector: _ -> [_ _ _ _ _ _ _ _ _ _]
      dyn-events: _ -> [_ _ _ _ _ _ _ _ _ _]
      timeout: _ -> [_ _ _ _ _ _ _ _ _ _]
      tunnel: w38 -> [_ w39 _ _ w54 w58 w62 _ _ _]
      event Timeout {
        n32 = event-data() -> ()  [unwired: 1 in, 2 out]
      }
      event "Init Trigger": Value Change {
        n33 = event-data() -> ()  [unwired: 1 in, 5 out]
        n34 = case shown="True" "Init Trigger" {
          tunnel: w39 -> [_ w42]
          frame False {
          }
          frame True {
            n35 = Enqueue Element(queue=w42, element=SpectrometerEvents."Init Button") -> ()  [unwired: 2 in, 3 out]
          }
        }
      }
      event "Spectrum": Mouse Down {
        n36 = event-data() -> ("Button"=w43:u16)  [unwired: 1 in, 4 out]
        n37 = case shown="2" w43 {
          frame 0, Default {
          }
          frame 2 {
            n38 = property on="Spectrum" class="XYGraph (strict)"() -> ("XScale.Minimum"=w49:dbl, "XScale.Maximum"=w48:dbl, "YScale.Minimum"=w47:dbl, "YScale.Maximum"=w46:dbl)  [unwired: 2 in, 2 out]
            n39 = call "getCenter.vi"("ymax"=w46, "ymin"=w47, "xmax"=w48, "xmin"=w49) -> ("y"=w44:dbl, "x"=w45:dbl)  [unwired: 6 in]
            n40 = property on="Spectrum" class="XYGraph (strict)"("Cursor.Cursor X"=w45, "Cursor.Cursor Y"=w44) -> ()  [unwired: 2 in, 2 out]
          }
        }
      }
      event "Spectrum": Cursor Move {
        n41 = event-data() -> ("CursLoc"=w52:cluster{"X":dbl, "Y":dbl})  [unwired: 1 in, 7 out]
        n42 = Unbundle By Name(w52) -> ("X"=→"Wavelength":dbl, "Y"=→"Intensity":dbl)
      }
      event "Continuous": Value Change {
        n43 = event-data() -> ()  [unwired: 1 in, 5 out]
        n44 = case shown="True" "Continuous" {
          tunnel: w54 -> [_ w56]
          frame False {
          }
          frame True {
            n45 = Enqueue Element(queue=w56, element=SpectrometerEvents."Acquire") -> ()  [unwired: 2 in, 3 out]
          }
        }
      }
      event "Acquire Trigger": Value Change {
        n46 = event-data() -> ()  [unwired: 1 in, 5 out]
        n47 = case shown="False" "Acquire Trigger" {
          tunnel: w58 -> [_ w60]
          frame False {
          }
          frame True {
            n48 = Enqueue Element(queue=w60, element=SpectrometerEvents."Acquire") -> ()  [unwired: 2 in, 3 out]
          }
        }
      }
      event "Acquire Background": Value Change {
        n49 = event-data() -> ()  [unwired: 1 in, 5 out]
        n50 = case shown="True" "Acquire Background" {
          tunnel: w62 -> [_ w66]
          frame False {
          }
          frame True {
            n51 = Enqueue Element(queue=w66, element=SpectrometerEvents."TimeOut") -> (queue out=w64:refnum<queue>)  [unwired: 2 in, 2 out]
            n52 = Enqueue Element(queue=w64, element=SpectrometerEvents."Acquire Background") -> ()  [unwired: 2 in, 3 out]
          }
        }
      }
      event "Reset Graph": Value Change {
        n53 = event-data() -> ()  [unwired: 1 in, 5 out]
        n54 = case shown="True" "Reset Graph" {
          frame False {
          }
          frame True {
            n55 = global read "StellarNet Globals.vi" "Spectrometer Wavelengths (All)"() -> (w69:sgl[][])
            n56 = call "RescaleSpectrometerGraphX.vi"("Spectrometer wavelengths"=w69) -> ("Numeric"=w71:sgl)  [unwired: 9 in, 1 out]
            n57 = property on="Spectrum" class="XYGraph (strict)"("YScale.Maximum"=65536.0 ("Y Scale.Range:Maximum")) -> ()  [unwired: 2 in, 2 out]
            n58 = property on="Spectrum" class="XYGraph (strict)"("XScale.Maximum"=w71, "XScale.Minimum"=300.0 ("X Scale.Range:Minimum")) -> ()  [unwired: 2 in, 2 out]
          }
        }
      }
      event "20ms": Value Change {
        n59 = event-data() -> ()  [unwired: 1 in, 5 out]
        n60 = case shown="True" "20ms" {
          frame False {
          }
          frame True {
            n61 = property on="Integration Time (ms)" class="DigNum (strict)"("Value"=20 ("Integration Time (ms)")) -> ()  [unwired: 2 in, 2 out]
          }
        }
      }
      event "1000 ms": Value Change {
        n62 = event-data() -> ()  [unwired: 1 in, 5 out]
        n63 = case shown="True" "1000 ms" {
          frame False {
          }
          frame True {
            n64 = property on="Integration Time (ms)" class="DigNum (strict)"("Value"=1000 ("Integration Time (ms)")) -> ()  [unwired: 2 in, 2 out]
          }
        }
      }
    }
    n65 = local read "STOP"() -> (w37:bool)
  }
  n66 = global write "StellarNet Globals.vi" "SpectraWiz Events"(w5) -> ()
  n67 = while {
    shift-right: [w86] -> _
    shift-left: errorcluster {"status"=FALSE, "code"=0, "source"=""} ("Error\nCluster\nconstant") -> [w87]
    shift-right: [w85] -> _
    shift-left: dbl[][][] [] -> [w89]
    shift-right: [w84] -> _
    shift-left: string[][][] [] -> [w88]
    tunnel: w5 -> [w83]
    tunnel: w1 -> [_]
    i -> [w91]
    stop <- w92 stop-if-true
    n68 = global read "StellarNet Globals.vi" "Spectrometer Wavelengths (All)"() -> (w77:sgl[][])
    n69 = global read "StellarNet Globals.vi" "Spectral Channels"() -> (w78:i32[])
    n70 = local read "Array"() -> (w81:bool[])
    n71 = call "InitScan.vi"("Spectral Channels Bool"=w81, "Spectrometer wavelengths (All)"=w77, "Spectral Channels (All)"=w78) -> ("Spectrometer wavelengths (filtered)"=w79:sgl[][], "Spectral Channels (filtered)"=w80:i32[])  [unwired: 7 in]
    n72 = Dequeue Element(queue=w83) -> (queue out=w82:refnum<queue>, element=w90:T2)  [unwired: 2 in, 2 out]
    n73 = case shown="\"Acquire\"" w90 {
      tunnel: w80 -> [_ w118 w290 w400 w486 w573]
      tunnel: w89 -> [w95 w115 w287 _ _ _]
      tunnel: w88 -> [w96 w117 w289 _ _ _]
      tunnel: w87 -> [w94 w116 w288 _ _ _]
      tunnel: [w96 w114 w286 w404 w490 w577] -> w84
      tunnel: [w94 w109 w281 _ _ _] -> w86
      tunnel: [w95 w113 w285 dbl[][][] [] dbl[][][] [] dbl[][][] []] -> w85
      tunnel: w82 -> [_ w106 w278 _ _ _]
      tunnel: w79 -> [_ w101 w274 _ _ _]
      frame "TimeOut", Default {
      }
      frame "Acquire" {
        n74 = disable-structure shown="Enabled" {
          disable-tunnel: [w124 w125] -> w120
          disable-tunnel: w116 -> [w123 w125]
          frame Disabled {
            n75 = call "closeSWWindows.vi"("error in (no error)"=w123) -> ("error out"=w124:errorcluster)  [unwired: 10 in]
          }
          frame Enabled {
          }
        }
        n76 = global read "StellarNet Globals.vi" "Spectrometer data array sizes"() -> (w100:i32[])
        n77 = local read "Continuous"() -> (w107:bool)
        n78 = local read "Save paths"() -> (w119:path[])
        n79 = property on="Spectrum" class="XYGraph (strict)"("YScale.Minimum"=0.0 ("Y Scale.Range:Maximum")) -> ()  [unwired: 2 in, 2 out]
        n80 = global write "StellarNet Globals.vi" "Scan OK"(FALSE ("Scan OK")) -> ()
        n81 = for {
          tunnel: w120 -> [w152]
          tunnel: [w151] -> w108
          tunnel: w115 -> [w148]
          tunnel: [w150] -> w113 mode=indexing
          tunnel: w117 -> [w135]
          tunnel: [w149] -> w114 mode=indexing
          tunnel: [w146] -> w110 mode=indexing
          tunnel: w119 -> [w136] mode=indexing
          tunnel: w118 -> [w138] mode=indexing
          tunnel: [w143] -> w112
          tunnel: w101 -> [w142] mode=indexing
          tunnel: w100 -> [w139]
          tunnel: [w141] -> w104 mode=indexing
          tunnel: [w140] -> w105 mode=indexing
          tunnel: [TRUE ("Scan OK")] -> w98
          i -> [w133]
          n82 = Decrement(x=w138) -> (x-1=w131:i32)
          n83 = Index Array(array=w135, index (dim 0)=w133) -> (element=w134:string[][])  [unwired: 2 in]
          n84 = Index Array(array=w139, index=w131) -> (element=w137:i32)
          n85 = Index Array(array=w148, index (dim 0)=w131) -> (element=w147:dbl[][])  [unwired: 2 in]
          n86 = flat-sequence {
            tunnel: [w183] -> w151
            tunnel: [w180] -> w150
            tunnel: w152 -> [w184]
            tunnel: w147 -> [w181]
            tunnel: w134 -> [w178]
            tunnel: [w179] -> w149
            tunnel: [w177] -> w146
            tunnel: w136 -> [w176]
            tunnel: w138 -> [w161]
            tunnel: [w175] -> w143
            tunnel: w142 -> [w164]
            tunnel: w137 -> [w174]
            tunnel: [w166] -> w141
            tunnel: [w153] -> _
            tunnel: w133 -> [w167]
            tunnel: [w165] -> w140
            tunnel: w131 -> [w154]
            tunnel: w131 -> [w153]
            frame #0 {
              # "add save data here"
              n87 = local read "Background"() -> (w172:sgl[][])
              n88 = property on="Integration Time (ms)" class="DigNum (strict)"() -> ("Value"=w170:i32)  [unwired: 2 in, 2 out]
              n89 = property on="Number of Scans to Average" class="DigNum (strict)"() -> ("Value"=w171:i32)  [unwired: 2 in, 2 out]
              n90 = Index Array(array=w172, index (row)=w153) -> (element=w158:sgl[])  [unwired: 1 in]
              n91 = local read "Watts"() -> (w157:bool)
              n92 = Empty Array?(array=w158) -> (empty?=w173:bool)
              n93 = call "AdjustSettings.vi"("Averaging"=w171, "Integration Time (msec)"=w170) -> ("Spectrometer Settings"=w168:T4)  [unwired: 9 in]
              n94 = call "StellarNet Scan.vi"("Channel Settings"=w168, "error in (no error)"=w184, "Integration Time (msec)"=w170, "Spectral Channel"=w161) -> ("error out"=w183:errorcluster, "buffer out"=w169:sgl[])  [unwired: 4 in, 2 out]
              n95 = Array Subset(array=w169, length=w174) -> (w163:sgl[])  [unwired: 1 in]
              n96 = case shown="True" w173 {
                tunnel: w158 -> [w211 _]
                tunnel: [w209 w217] -> w155
                tunnel: w163 -> [w212 w217]
                frame False {
                  n97 = Subtract(x=w212, y=w211) -> (x-y=w210:sgl[])
                  n98 = for {
                    tunnel: w210 -> [w214] mode=indexing
                    tunnel: [w215] -> w209 mode=indexing
                    n99 = Greater Than 0?(x=w214) -> (x > 0?=w216:bool)
                    n100 = Select(t=w214, s=w216, f=sgl 0.0) -> (s? t:f=w215:sgl)
                  }
                }
                frame True {
                }
              }
              n101 = case shown="True" w157 {
                tunnel: [w188 w189] -> w156
                tunnel: w155 -> [w188 w191]
                tunnel: w154 -> [_ w192]
                frame False {
                }
                frame True {
                  n102 = call "CalibrationExtract.vi"("Channel"=w192) -> ("Calibration Values"=w190:dbl[])  [unwired: 10 in]
                  n103 = Compound Arithmetic op=MULTIPLY(w191, w190) -> (w189:dbl[])
                }
              }
              n104 = local read "Normalize"() -> (w159:bool)
              n105 = case shown="True" w159 {
                tunnel: [w193 w194] -> w160
                tunnel: w156 -> [w193 w195]
                frame False {
                }
                frame True {
                  n106 = call "Normalize.vi"("Input"=w195) -> ("Normalized"=w194:sgl[])  [unwired: 10 in]
                }
              }
              n107 = property on="Autosave" class="Bool (strict)"() -> ("Value"=w182:bool)  [unwired: 2 in, 2 out]
              n108 = Array Max & Min(array=w160) -> (max value=w186:dbl, max index (indices)=w187:i32)  [unwired: 2 out]
              n109 = Bundle("Spectrometer wavelengths (filtered)"=w164, "Normalized"=w160) -> (w166:T5)  [unwired: 1 in]
              n110 = global write "StellarNet Globals.vi" "Spectrum"(w166) -> ()
              n111 = case shown="True" "Enable fit" {
                tunnel: w160 -> [_ w199]
                tunnel: w167 -> [_ w198]
                tunnel: [_ w197] -> w165
                tunnel: w164 -> [_ w196]
                frame False {
                }
                frame True {
                  n112 = case shown="0" w198 {
                    tunnel: w199 -> [w204 _]
                    tunnel: [w208 _] -> w197
                    tunnel: w196 -> [w203 _]
                    frame 0 {
                      # "if 0 = black comet"
                      n113 = property on="Spectrum" class="XYGraph (strict)"() -> ("Cursor.Cursor Y"=w200:dbl)  [unwired: 2 in, 2 out]
                      n114 = property on="Spectrum" class="XYGraph (strict)"() -> ("Cursor.Cursor X"=w207:dbl)  [unwired: 2 in, 2 out]
                      n115 = call "FitGaussian.vi"("X"=w203, "Y"=w204, "Amplitude fit"=w200, "Initial X"=w207, "FWHM"="FWHM", "Offset"="Offset") -> ("Fit Spectrum"=w208:cluster{sgl[], "Best Gaussian Fit":dbl[]}, "center"=→"Center (nm)":dbl, "FWHM"=→"FWHM":dbl)  [unwired: 5 in, 2 out]
                    }
                    frame 1, Default {
                    }
                  }
                }
              }
              n116 = case shown="True" w182 {
                tunnel: w160 -> [w223 w247]
                tunnel: w181 -> [w221 w246]
                tunnel: [w222 _] -> w180
                tunnel: w178 -> [w220 w245]
                tunnel: [w219 _] -> w179
                tunnel: w176 -> [w218 _]
                frame True {
                  n117 = disable-structure shown="Enabled" {
                    disable-tunnel: w223 -> [w232 w244]
                    disable-tunnel: [w227 w241] -> w222
                    disable-tunnel: w221 -> [w225 w243]
                    disable-tunnel: w220 -> [_ w235]
                    disable-tunnel: [_ w233] -> w219
                    disable-tunnel: w218 -> [_ w237]
                    frame Disabled {
                      n118 = global read "GlobalUI.vi" "Stage Position (mm)"() -> (w224:dbl)
                      n119 = Build Array (concatenate)(w224, w232) -> (w231:dbl[])
                      n120 = Build Array (concatenate)(w225, w231) -> (w227:dbl[][])
                      n121 = local read item#-1() -> (w226)
                      n122 = call-poly <vilib>:"Write To Spreadsheet File.vi"("delimiter (\\t)"="," ("delimiter (\\t)"), "transpose? (no:F)"=TRUE, "append to file? (new file:F)"=FALSE, "2D data"=w227, "file path (dialog if empty)"=w226) -> ()  [unwired: 3 in, 1 out]
                    }
                    frame Enabled {
                      n123 = global read "GlobalUI.vi" "Stage Position (mm)"() -> (w242:dbl)
                      n124 = Build Array (concatenate)(w242, w244) -> (w239:dbl[])
                      n125 = Build Array (concatenate)(w243, w239) -> (w241:dbl[][])
                      n126 = Number To Fractional String(number=w239, precision (6)=i16 3) -> (F-format string=w234:string[])  [unwired: 2 in]
                      n127 = Build Array (concatenate)(w235, w234) -> (w233:string[][])
                      n128 = call-poly <vilib>:"Write To Spreadsheet File.vi"("delimiter (\\t)"="," ("delimiter (\\t)"), "transpose? (no:F)"=TRUE, "2D data"=w233, "file path (dialog if empty)"=w237) -> ()  [unwired: 4 in, 1 out]
                    }
                  }
                }
                frame False {
                  n129 = disable-structure shown="Enabled" {
                    disable-tunnel: w247 -> [w256 w267]
                    disable-tunnel: [w251 w264] -> _
                    disable-tunnel: w246 -> [w249 w266]
                    disable-tunnel: w245 -> [_ w261]
                    disable-tunnel: [_ w257] -> _
                    frame Disabled {
                      n130 = global read "GlobalUI.vi" "Stage Position (mm)"() -> (w248:dbl)
                      n131 = Build Array (concatenate)(w248, w256) -> (w255:dbl[])
                      n132 = Build Array (concatenate)(w249, w255) -> (w251:dbl[][])
                      n133 = local read item#-1() -> (w250)
                      n134 = call-poly <vilib>:"Write To Spreadsheet File.vi"("delimiter (\\t)"="," ("delimiter (\\t)"), "transpose? (no:F)"=TRUE, "append to file? (new file:F)"=FALSE, "2D data"=w251, "file path (dialog if empty)"=w250) -> ()  [unwired: 3 in, 1 out]
                    }
                    frame Enabled {
                      n135 = Transpose 2D Array(2D array=w261) -> (transposed array=w260:string[][])
                      n136 = global read "GlobalUI.vi" "Stage Position (mm)"() -> (w265:dbl)
                      n137 = Build Array (concatenate)(w265, w267) -> (w262:dbl[])
                      n138 = Build Array (concatenate)(w266, w262) -> (w264:dbl[][])
                      n139 = Number To Fractional String(number=w262, precision (6)=i16 3) -> (F-format string=w259:string[])  [unwired: 2 in]
                      n140 = Build Array (concatenate)(w260, w259) -> (w258:string[][])
                      n141 = Transpose 2D Array(2D array=w258) -> (transposed array=w257:string[][])
                    }
                  }
                }
              }
              n142 = Index Array(array=w164, index=w187) -> (element=w185:sgl)
              n143 = Bundle(w186, "lamda"=w185) -> (w177:cluster{dbl, "lamda":sgl})  [unwired: 1 in]
              n144 = Tick Count (ms)() -> (millisecond timer value=w175:u32)
            }
          }
          n145 = property on="Integration Time (ms)" class="DigNum (strict)"() -> ("Value"=w144:i32)  [unwired: 2 in, 2 out]
          n146 = property on="Number of Scans to Average" class="DigNum (strict)"() -> ("Value"=w145:i32)  [unwired: 2 in, 2 out]
          n147 = global write "StellarNet Globals.vi" "Integration Time (ms)"(w144) -> ()
          n148 = global write "StellarNet Globals.vi" "Number of Scans to Average"(w145) -> ()
        }
        n149 = Tick Count (ms)() -> (millisecond timer value=w111:u32)
        n150 = case shown="True" w107 {
          tunnel: [w126 w127] -> w109
          tunnel: w108 -> [w126 w128]
          tunnel: w106 -> [_ w129]
          frame False {
          }
          frame True {
            n151 = Enqueue Element(queue=w129, element=SpectrometerEvents."Acquire", error in (no error)=w128) -> (error out=w127:errorcluster)  [unwired: 1 in, 2 out]
          }
        }
        n152 = Build Array (concatenate)(w104, w105) -> (w103:T6)
        n153 = local write "Spectral history"(w110) -> ()
        n154 = local write "Spectrum"(w103) -> ()
        n155 = global write "StellarNet Globals.vi" "Scan OK"(w98) -> ()
        n156 = Subtract(x=w112, y=w111) -> (x-y=w99:u32)
        n157 = local write "time elapsed prev scan (ms)"(w99) -> ()
        n158 = disable-structure shown="Disabled" {
          disable-tunnel: w103 -> [w122 _]
          frame Disabled {
            n159 = call "RescaleSpectrometerGraph.vi"("Array"=w122) -> ("Ymax"=w121:dbl)  [unwired: 10 in]
            n160 = property on="Spectrum" class="XYGraph (strict)"("YScale.Maximum"=w121) -> ()  [unwired: 2 in, 2 out]
          }
          frame Enabled {
          }
        }
        n161 = global write "StellarNet Globals.vi" "time elapsed on previous scan (ms)"(w99) -> ()
      }
      frame "Acquire Background" {
        n162 = disable-structure shown="Enabled" {
          disable-tunnel: [w294 w295] -> w292
          disable-tunnel: w288 -> [w293 w295]
          frame Disabled {
            n163 = call "closeSWWindows.vi"("error in (no error)"=w293) -> ("error out"=w294:errorcluster)  [unwired: 10 in]
          }
          frame Enabled {
          }
        }
        n164 = global read "StellarNet Globals.vi" "Spectrometer data array sizes"() -> (w273:i32[])
        n165 = local read "Continuous"() -> (w279:bool)
        n166 = local read "Save paths"() -> (w291:path[])
        n167 = property on="Spectrum" class="XYGraph (strict)"("YScale.Minimum"=0.0 ("Y Scale.Range:Maximum")) -> ()  [unwired: 2 in, 2 out]
        n168 = global write "StellarNet Globals.vi" "Scan OK"(FALSE ("Scan OK")) -> ()
        n169 = for {
          tunnel: w292 -> [w322]
          tunnel: [w321] -> w280
          tunnel: w287 -> [w318]
          tunnel: [w320] -> w285 mode=indexing
          tunnel: w289 -> [w306]
          tunnel: [w319] -> w286 mode=indexing
          tunnel: [w316] -> w282 mode=indexing
          tunnel: w291 -> [w307] mode=indexing
          tunnel: w290 -> [w309] mode=indexing
          tunnel: [w313] -> w284
          tunnel: w274 -> [w312] mode=indexing
          tunnel: w273 -> [w310]
          tunnel: [w311] -> w269 mode=indexing
          tunnel: [TRUE ("Scan OK")] -> w271
          tunnel: [w301] -> w268 mode=indexing
          i -> [w303]
          n170 = Decrement(x=w309) -> (x-1=w305:i32)
          n171 = Index Array(array=w306, index (dim 0)=w303) -> (element=w304:string[][])  [unwired: 2 in]
          n172 = Index Array(array=w310, index=w305) -> (element=w308:i32)
          n173 = Index Array(array=w318, index (dim 0)=w305) -> (element=w317:dbl[][])  [unwired: 2 in]
          n174 = flat-sequence {
            tunnel: [w342] -> w321
            tunnel: [w339] -> w320
            tunnel: w322 -> [w343]
            tunnel: w317 -> [w340]
            tunnel: w304 -> [w337]
            tunnel: [w338] -> w319
            tunnel: [w336] -> w316
            tunnel: w307 -> [w335]
            tunnel: w309 -> [w326]
            tunnel: [w334] -> w313
            tunnel: w312 -> [w324]
            tunnel: w308 -> [w333]
            tunnel: [w328] -> w311
            tunnel: w303 -> [_]
            tunnel: w303 -> [_]
            tunnel: [w323] -> w301
            frame #0 {
              # "add save data here"
              n175 = property on="Integration Time (ms)" class="DigNum (strict)"() -> ("Value"=w331:i32)  [unwired: 2 in, 2 out]
              n176 = property on="Number of Scans to Average" class="DigNum (strict)"() -> ("Value"=w332:i32)  [unwired: 2 in, 2 out]
              n177 = call "AdjustSettings.vi"("Averaging"=w332, "Integration Time (msec)"=w331) -> ("Spectrometer Settings"=w329:T4)  [unwired: 9 in]
              n178 = call "StellarNet Scan.vi"("Channel Settings"=w329, "error in (no error)"=w343, "Integration Time (msec)"=w331, "Spectral Channel"=w326) -> ("error out"=w342:errorcluster, "buffer out"=w330:sgl[])  [unwired: 4 in, 2 out]
              n179 = Array Subset(array=w330, length=w333) -> (w327:sgl[])  [unwired: 1 in]
              n180 = local read "Normalize"() -> (w325:bool)
              n181 = case shown="False" w325 {
                tunnel: w327 -> [w347 w349]
                tunnel: [w347 w348] -> w323
                frame False {
                }
                frame True {
                  n182 = call "Normalize.vi"("Input"=w349) -> ("Normalized"=w348:sgl[])  [unwired: 10 in]
                }
              }
              n183 = property on="Autosave" class="Bool (strict)"() -> ("Value"=w341:bool)  [unwired: 2 in, 2 out]
              n184 = Array Max & Min(array=w323) -> (max value=w345:sgl, max index (indices)=w346:i32)  [unwired: 2 out]
              n185 = Bundle("Spectrometer wavelengths (filtered)"=w324, "Normalized"=w323) -> (w328:T7)  [unwired: 1 in]
              n186 = global write "StellarNet Globals.vi" "Spectrum"(w328) -> ()
              n187 = case shown="True" w341 {
                tunnel: w323 -> [w355 w379]
                tunnel: w340 -> [w353 w378]
                tunnel: [w354 _] -> w339
                tunnel: w337 -> [w352 w377]
                tunnel: [w351 _] -> w338
                tunnel: w335 -> [w350 _]
                frame True {
                  n188 = disable-structure shown="Enabled" {
                    disable-tunnel: w355 -> [w364 w376]
                    disable-tunnel: [w359 w373] -> w354
                    disable-tunnel: w353 -> [w357 w375]
                    disable-tunnel: w352 -> [_ w367]
                    disable-tunnel: [_ w365] -> w351
                    disable-tunnel: w350 -> [_ w369]
                    frame Disabled {
                      n189 = global read "GlobalUI.vi" "Stage Position (mm)"() -> (w356:dbl)
                      n190 = Build Array (concatenate)(w356, w364) -> (w363:dbl[])
                      n191 = Build Array (concatenate)(w357, w363) -> (w359:dbl[][])
                      n192 = local read item#-1() -> (w358)
                      n193 = call-poly <vilib>:"Write To Spreadsheet File.vi"("delimiter (\\t)"="," ("delimiter (\\t)"), "transpose? (no:F)"=TRUE, "append to file? (new file:F)"=FALSE, "2D data"=w359, "file path (dialog if empty)"=w358) -> ()  [unwired: 3 in, 1 out]
                    }
                    frame Enabled {
                      n194 = global read "GlobalUI.vi" "Stage Position (mm)"() -> (w374:dbl)
                      n195 = Build Array (concatenate)(w374, w376) -> (w371:dbl[])
                      n196 = Build Array (concatenate)(w375, w371) -> (w373:dbl[][])
                      n197 = Number To Fractional String(number=w371, precision (6)=i16 3) -> (F-format string=w366:string[])  [unwired: 2 in]
                      n198 = Build Array (concatenate)(w367, w366) -> (w365:string[][])
                      n199 = call-poly <vilib>:"Write To Spreadsheet File.vi"("delimiter (\\t)"="," ("delimiter (\\t)"), "transpose? (no:F)"=TRUE, "2D data"=w365, "file path (dialog if empty)"=w369) -> ()  [unwired: 4 in, 1 out]
                    }
                  }
                }
                frame False {
                  n200 = disable-structure shown="Enabled" {
                    disable-tunnel: w379 -> [w388 w399]
                    disable-tunnel: [w383 w396] -> _
                    disable-tunnel: w378 -> [w381 w398]
                    disable-tunnel: w377 -> [_ w393]
                    disable-tunnel: [_ w389] -> _
                    frame Disabled {
                      n201 = global read "GlobalUI.vi" "Stage Position (mm)"() -> (w380:dbl)
                      n202 = Build Array (concatenate)(w380, w388) -> (w387:dbl[])
                      n203 = Build Array (concatenate)(w381, w387) -> (w383:dbl[][])
                      n204 = local read item#-1() -> (w382)
                      n205 = call-poly <vilib>:"Write To Spreadsheet File.vi"("delimiter (\\t)"="," ("delimiter (\\t)"), "transpose? (no:F)"=TRUE, "append to file? (new file:F)"=FALSE, "2D data"=w383, "file path (dialog if empty)"=w382) -> ()  [unwired: 3 in, 1 out]
                    }
                    frame Enabled {
                      n206 = Transpose 2D Array(2D array=w393) -> (transposed array=w392:string[][])
                      n207 = global read "GlobalUI.vi" "Stage Position (mm)"() -> (w397:dbl)
                      n208 = Build Array (concatenate)(w397, w399) -> (w394:dbl[])
                      n209 = Build Array (concatenate)(w398, w394) -> (w396:dbl[][])
                      n210 = Number To Fractional String(number=w394, precision (6)=i16 3) -> (F-format string=w391:string[])  [unwired: 2 in]
                      n211 = Build Array (concatenate)(w392, w391) -> (w390:string[][])
                      n212 = Transpose 2D Array(2D array=w390) -> (transposed array=w389:string[][])
                    }
                  }
                }
              }
              n213 = Index Array(array=w324, index=w346) -> (element=w344:sgl)
              n214 = Bundle(w345, "lamda"=w344) -> (w336:cluster{sgl, "lamda":sgl})  [unwired: 1 in]
              n215 = Tick Count (ms)() -> (millisecond timer value=w334:u32)
            }
          }
          n216 = property on="Integration Time (ms)" class="DigNum (strict)"() -> ("Value"=w314:i32)  [unwired: 2 in, 2 out]
          n217 = property on="Number of Scans to Average" class="DigNum (strict)"() -> ("Value"=w315:i32)  [unwired: 2 in, 2 out]
          n218 = global write "StellarNet Globals.vi" "Integration Time (ms)"(w314) -> ()
          n219 = global write "StellarNet Globals.vi" "Number of Scans to Average"(w315) -> ()
        }
        n220 = Tick Count (ms)() -> (millisecond timer value=w283:u32)
        n221 = case shown="False" w279 {
          tunnel: [w296 w297] -> w281
          tunnel: w280 -> [w296 w298]
          tunnel: w278 -> [_ w299]
          frame False {
          }
          frame True {
            n222 = Enqueue Element(queue=w299, element=SpectrometerEvents."Acquire", error in (no error)=w298) -> (error out=w297:errorcluster)  [unwired: 1 in, 2 out]
          }
        }
        n223 = local write "Spectral history"(w282) -> ()
        n224 = local write "Spectrum"(w269) -> ()
        n225 = global write "StellarNet Globals.vi" "Scan OK"(w271) -> ()
        n226 = Subtract(x=w284, y=w283) -> (x-y=w272:u32)
        n227 = local write "Background"(w268) -> ()
        n228 = call "RescaleSpectrometerGraph.vi"("Previous Ymax"=0.0, "Array"=w269) -> ("Ymax"=w277:dbl)  [unwired: 9 in]
        n229 = local write "time elapsed prev scan (ms)"(w272) -> ()
        n230 = property on="Spectrum" class="XYGraph (strict)"("YScale.Maximum"=w277) -> ()  [unwired: 2 in, 2 out]
        n231 = global write "StellarNet Globals.vi" "time elapsed on previous scan (ms)"(w272) -> ()
      }
      frame "Init Button" {
        n232 = global read "StellarNet Globals.vi" "Spectrometer wavelengths (string)"() -> (w401:string[][])
        n233 = for {
          tunnel: [w413] -> w404 mode=indexing
          tunnel: w400 -> [w406] mode=indexing
          tunnel: [w411] -> w403 mode=indexing
          tunnel: w401 -> [w408]
          n234 = Decrement(x=w406) -> (x-1=w405:i32)
          n235 = Index Array(array=w408, index (row)=w405) -> (element=w407:string[])  [unwired: 1 in]
          n236 = flat-sequence {
            tunnel: [w425] -> w415
            tunnel: [w423] -> w414
            tunnel: w406 -> [w419]
            tunnel: [w419] -> w412
            tunnel: [w422] -> w410
            tunnel: w407 -> [w422]
            tunnel: [w420] -> w409
            tunnel: w405 -> [w416]
            tunnel: [w467] -> _
            tunnel: w415 -> [w465]
            tunnel: w414 -> [_]
            tunnel: [w466] -> w413
            tunnel: w412 -> [w467]
            tunnel: [w464] -> w411
            tunnel: w410 -> [w463]
            tunnel: w409 -> [_]
            frame #0 {
              w423 = cluster{sgl, "lamda":sgl}[] []  # Empty array
              n237 = Number To Fractional String(number=w419, precision (6)=i16 0) -> (F-format string=w417:string)  [unwired: 2 in]
              n238 = disable-structure shown="Enabled" {
                disable-tunnel: [w433 w442] -> w424
                disable-tunnel: [w430 _] -> w421
                disable-tunnel: w417 -> [w428 w441]
                disable-tunnel: w416 -> [_ w445]
                frame Enabled {
                  n239 = global read "GlobalUI.vi" "Save Path"() -> (w431:path)
                  n240 = Concatenate Strings("ch" ("string"), w428) -> (w427:string)
                  n241 = flat-sequence {
                    tunnel: [w440] -> w426
                    frame #0 {
                      n242 = global write "GlobalUI.vi" "Sample Description"("File Description") -> ()
                      n243 = global write "GlobalUI.vi" "Filenaming Mode"(Filenaming."Just Description" ("Filenaming Mode")) -> ()
                    }
                    frame #1 {
                      n244 = call "naming.vi"() -> ("filename"=w440:string)  [unwired: 15 in]
                    }
                  }
                  n245 = call "addTimeToPath.vi"("Path"=w431) -> ("Time Path (Path)"=w430:path)  [unwired: 9 in, 1 out]
                  n246 = Path To String(path=w430) -> (string=w436:string)
                  n247 = Concatenate Strings(w436, "\\" ("string"), w426, w427) -> (w432:string)
                  n248 = Concatenate Strings(w432, "_s_00.csv" ("string")) -> (w434:string)
                  n249 = String To Path(string=w434) -> (path=w433:path)
                }
                frame Disabled {
                  n250 = local read "Save paths"() -> (w446:path[])
                  n251 = Index Array(array=w446, index=w445) -> (element=w443:path)
                  n252 = Path Type(1:w443) -> (0:w444:i16)
                  n253 = case shown="2" w444 {
                    tunnel: w443 -> [w447 _]
                    tunnel: [w447 w448] -> w442
                    tunnel: w441 -> [_ w451]
                    frame 0, Default {
                    }
                    frame 2 {
                      n254 = call <vilib>:"Dflt Data Dir.vi"() -> ("App:Default Data Directory"=w456:path)
                      n255 = Path To String(path=w456) -> (string=w455:string)
                      n256 = Concatenate Strings(w455, "Spectrometer" ("string"), "ch" ("string"), w451) -> (w453:string)
                      n257 = Concatenate Strings(w453, "_00.csv" ("string")) -> (w449:string)
                      n258 = String To Path(string=w449) -> (path=w448:path)
                    }
                  }
                }
              }
              n259 = property on="Spectral history" class="WFChart (strict)"("History Data"=w423) -> ()  [unwired: 2 in, 2 out]
              n260 = Create Folder(path (use dialog)=w421) -> (error out=w420:errorcluster)  [unwired: 2 in, 2 out]
              n261 = call "fixfilename.vi"("Path"=w424) -> ("fixed path"=w425:path)  [unwired: 9 in, 1 out]
            }
            frame #1 {
              n262 = Build Array(w463) -> (w460:string[][])
              n263 = Insert Into Array(array=w460, index (col)=0 ("disabled index (col)"), new element=string[][] [[" "]] ("element")) -> (w457:string[][])  [unwired: 1 in]
              n264 = property on="Autosave" class="Bool (strict)"() -> ("Value"=w462:bool)  [unwired: 2 in, 2 out]
              n265 = case shown="True" w462 {
                tunnel: w465 -> [w468 w472]
                tunnel: [w469 w471] -> w466
                tunnel: w457 -> [w469 w471]
                tunnel: [w468 w470] -> w464
                frame False {
                }
                frame True {
                  n266 = disable-structure shown="Enabled" {
                    disable-tunnel: w472 -> [w473 w483]
                    disable-tunnel: w471 -> [_ w485]
                    disable-tunnel: [_ w483] -> w470
                    frame Disabled {
                      n267 = Write to Text File(file (use dialog)=w473) -> ()  [unwired: 3 in, 3 out]
                      n268 = Concatenate Strings("," ("delimiter (Tab)"), "\r") -> (w476:string)
                      n269 = Array To Spreadsheet String(delimiter (Tab)=w476, 3:"%.3f" ("format string")) -> (spreadsheet string=w480:string)  [unwired: 1 in]
                      n270 = Concatenate Strings("," ("string"), "\r", w480) -> (w479:string)
                      n271 = Build Array(w479) -> ()  [unwired: 1 out]
                    }
                    frame Enabled {
                      n272 = call-poly <vilib>:"Write To Spreadsheet File.vi"("transpose? (no:F)"=TRUE, "format (%s)"="%.7f", "2D data"=w485, "file path (dialog if empty)"=w483) -> ()  [unwired: 4 in, 1 out]
                    }
                  }
                }
              }
              n273 = global write "GlobalUI.vi" "SW Initializing"(FALSE ("SW Initializing")) -> ()
            }
          }
        }
        n274 = local write "Save paths"(w403) -> ()
      }
      frame "Init Background" {
        n275 = global read "StellarNet Globals.vi" "Spectrometer wavelengths (string)"() -> (w487:string[][])
        n276 = for {
          tunnel: [w499] -> w490 mode=indexing
          tunnel: w486 -> [w492] mode=indexing
          tunnel: [w497] -> w489 mode=indexing
          tunnel: w487 -> [w494]
          n277 = Decrement(x=w492) -> (x-1=w491:i32)
          n278 = Index Array(array=w494, index (row)=w491) -> (element=w493:string[])  [unwired: 1 in]
          n279 = flat-sequence {
            tunnel: [w511] -> w501
            tunnel: [w509] -> w500
            tunnel: w492 -> [w505]
            tunnel: [w505] -> w498
            tunnel: [w508] -> w496
            tunnel: w493 -> [w508]
            tunnel: [w506] -> w495
            tunnel: w491 -> [w502]
            tunnel: [w554] -> _
            tunnel: w501 -> [w552]
            tunnel: w500 -> [_]
            tunnel: [w553] -> w499
            tunnel: w498 -> [w554]
            tunnel: [w551] -> w497
            tunnel: w496 -> [w550]
            tunnel: w495 -> [_]
            frame #0 {
              w509 = cluster{sgl, "lamda":sgl}[] []  # Empty array
              n280 = Number To Fractional String(number=w505, precision (6)=i16 0) -> (F-format string=w503:string)  [unwired: 2 in]
              n281 = disable-structure shown="Enabled" {
                disable-tunnel: [w520 w529] -> w510
                disable-tunnel: [w517 _] -> w507
                disable-tunnel: w503 -> [w515 w528]
                disable-tunnel: w502 -> [_ w532]
                frame Enabled {
                  n282 = global read "GlobalUI.vi" "Save Path"() -> (w518:path)
                  n283 = Concatenate Strings("ch" ("string"), w515) -> (w514:string)
                  n284 = flat-sequence {
                    tunnel: [w527] -> w513
                    frame #0 {
                      n285 = local read "File Description"() -> (w525:string)
                      n286 = global write "GlobalUI.vi" "Sample Description"(w525) -> ()
                      n287 = global write "GlobalUI.vi" "Filenaming Mode"(Filenaming."Just Description" ("Filenaming Mode")) -> ()
                    }
                    frame #1 {
                      n288 = call "naming.vi"() -> ("filename"=w527:string)  [unwired: 15 in]
                    }
                  }
                  n289 = call "addTimeToPath.vi"("Path"=w518) -> ("Time Path (Path)"=w517:path)  [unwired: 9 in, 1 out]
                  n290 = Path To String(path=w517) -> (string=w523:string)
                  n291 = Concatenate Strings(w523, "\\" ("string"), w513, w514, "_background" ("string")) -> (w519:string)
                  n292 = Concatenate Strings(w519, "_s_00.csv" ("string")) -> (w521:string)
                  n293 = String To Path(string=w521) -> (path=w520:path)
                }
                frame Disabled {
                  n294 = local read "Save paths"() -> (w533:path[])
                  n295 = Index Array(array=w533, index=w532) -> (element=w530:path)
                  n296 = Path Type(1:w530) -> (0:w531:i16)
                  n297 = case shown="2" w531 {
                    tunnel: w530 -> [w534 _]
                    tunnel: [w534 w535] -> w529
                    tunnel: w528 -> [_ w538]
                    frame 0, Default {
                    }
                    frame 2 {
                      n298 = call <vilib>:"Dflt Data Dir.vi"() -> ("App:Default Data Directory"=w543:path)
                      n299 = Path To String(path=w543) -> (string=w542:string)
                      n300 = Concatenate Strings(w542, "Spectrometer" ("string"), "ch" ("string"), w538) -> (w540:string)
                      n301 = Concatenate Strings(w540, "_00.csv" ("string")) -> (w536:string)
                      n302 = String To Path(string=w536) -> (path=w535:path)
                    }
                  }
                }
              }
              n303 = property on="Spectral history" class="WFChart (strict)"("History Data"=w509) -> ()  [unwired: 2 in, 2 out]
              n304 = Create Folder(path (use dialog)=w507) -> (error out=w506:errorcluster)  [unwired: 2 in, 2 out]
              n305 = call "fixfilename.vi"("Path"=w510) -> ("fixed path"=w511:path)  [unwired: 9 in, 1 out]
            }
            frame #1 {
              n306 = Build Array(w550) -> (w547:string[][])
              n307 = Insert Into Array(array=w547, index (col)=0 ("disabled index (col)"), new element=string[][] [[" "]] ("element")) -> (w544:string[][])  [unwired: 1 in]
              n308 = property on="Autosave" class="Bool (strict)"() -> ("Value"=w549:bool)  [unwired: 2 in, 2 out]
              n309 = case shown="True" w549 {
                tunnel: w552 -> [w555 w559]
                tunnel: [w556 w558] -> w553
                tunnel: w544 -> [w556 w558]
                tunnel: [w555 w557] -> w551
                frame False {
                }
                frame True {
                  n310 = disable-structure shown="Enabled" {
                    disable-tunnel: w559 -> [w560 w570]
                    disable-tunnel: w558 -> [_ w572]
                    disable-tunnel: [_ w570] -> w557
                    frame Disabled {
                      n311 = Write to Text File(file (use dialog)=w560) -> ()  [unwired: 3 in, 3 out]
                      n312 = Concatenate Strings("," ("delimiter (Tab)"), "\r") -> (w563:string)
                      n313 = Array To Spreadsheet String(delimiter (Tab)=w563, 3:"%.3f" ("format string")) -> (spreadsheet string=w567:string)  [unwired: 1 in]
                      n314 = Concatenate Strings("," ("string"), "\r", w567) -> (w566:string)
                      n315 = Build Array(w566) -> ()  [unwired: 1 out]
                    }
                    frame Enabled {
                      n316 = call-poly <vilib>:"Write To Spreadsheet File.vi"("transpose? (no:F)"=TRUE, "format (%s)"="%.7f", "2D data"=w572, "file path (dialog if empty)"=w570) -> ()  [unwired: 4 in, 1 out]
                    }
                  }
                }
              }
              n317 = global write "GlobalUI.vi" "SW Initializing"(FALSE ("SW Initializing")) -> ()
            }
          }
        }
        n318 = local write "Save paths"(w489) -> ()
      }
      frame "Init Programmatically" {
        n319 = global read "StellarNet Globals.vi" "Spectrometer wavelengths (string)"() -> (w574:string[][])
        n320 = for {
          tunnel: [w586] -> w577 mode=indexing
          tunnel: w573 -> [w580] mode=indexing
          tunnel: [w584] -> w576 mode=indexing
          tunnel: w574 -> [w582]
          n321 = Decrement(x=w580) -> (x-1=w579:i32)
          n322 = Index Array(array=w582, index (row)=w579) -> (element=w581:string[])  [unwired: 1 in]
          n323 = flat-sequence {
            tunnel: [w592] -> w588
            tunnel: [w607] -> w587
            tunnel: w580 -> [w605]
            tunnel: [w605] -> w585
            tunnel: [w606] -> w583
            tunnel: w581 -> [w606]
            tunnel: w579 -> [w591]
            tunnel: [w589] -> w578
            tunnel: [w618] -> _
            tunnel: w588 -> [w616]
            tunnel: w587 -> [_]
            tunnel: [w617] -> w586
            tunnel: w585 -> [w618]
            tunnel: [w615] -> w584
            tunnel: w583 -> [w614]
            tunnel: w578 -> [_]
            frame #0 {
              w607 = cluster{sgl, "lamda":sgl}[] []  # Empty array
              n324 = Number To Fractional String(number=w591, precision (6)=i16 0) -> (F-format string=w594:string)  [unwired: 2 in]
              n325 = global read "GlobalUI.vi" "Save Path"() -> (w597:path)
              n326 = Concatenate Strings("ch" ("string"), w594) -> (w593:string)
              n327 = property on="Spectral history" class="WFChart (strict)"("History Data"=w607) -> ()  [unwired: 2 in, 2 out]
              n328 = call "addTimeToPath.vi"("Path"=w597) -> ("Time Path (Path)"=w596:path)  [unwired: 9 in, 1 out]
              n329 = call "naming.vi"() -> ("filename"=w598:string)  [unwired: 15 in]
              n330 = Path To String(path=w596) -> (string=w603:string)
              n331 = Concatenate Strings(w603, "\\" ("string"), w598, w593) -> (w599:string)
              n332 = Concatenate Strings(w599, "_s_00.csv" ("string")) -> (w601:string)
              n333 = String To Path(string=w601) -> (path=w600:path)
              n334 = Create Folder(path (use dialog)=w596) -> (error out=w589:errorcluster)  [unwired: 2 in, 2 out]
              n335 = call "fixfilename.vi"("Path"=w600) -> ("fixed path"=w592:path)  [unwired: 9 in, 1 out]
            }
            frame #1 {
              n336 = disable-structure shown="Disabled" {
                frame Disabled {
                  n337 = local write "Background"(dbl[][] [] ("Background")) -> ()
                }
                frame Enabled {
                }
              }
              n338 = Build Array(w614) -> (w611:string[][])
              n339 = Insert Into Array(array=w611, index (col)=0 ("disabled index (col)"), new element=string[][] [[" "]] ("element")) -> (w608:string[][])  [unwired: 1 in]
              n340 = property on="Autosave" class="Bool (strict)"() -> ("Value"=w613:bool)  [unwired: 2 in, 2 out]
              n341 = case shown="True" w613 {
                tunnel: w616 -> [w620 w624]
                tunnel: [w621 w623] -> w617
                tunnel: w608 -> [w621 w623]
                tunnel: [w620 w622] -> w615
                frame False {
                }
                frame True {
                  n342 = disable-structure shown="Enabled" {
                    disable-tunnel: w624 -> [w625 w635]
                    disable-tunnel: w623 -> [_ w637]
                    disable-tunnel: [_ w635] -> w622
                    frame Disabled {
                      n343 = Write to Text File(file (use dialog)=w625) -> ()  [unwired: 3 in, 3 out]
                      n344 = Concatenate Strings("," ("delimiter (Tab)"), "\r") -> (w628:string)
                      n345 = Array To Spreadsheet String(delimiter (Tab)=w628, 3:"%.3f" ("format string")) -> (spreadsheet string=w632:string)  [unwired: 1 in]
                      n346 = Concatenate Strings("," ("string"), "\r", w632) -> (w631:string)
                      n347 = Build Array(w631) -> ()  [unwired: 1 out]
                    }
                    frame Enabled {
                      n348 = call-poly <vilib>:"Write To Spreadsheet File.vi"("transpose? (no:F)"=TRUE, "format (%s)"="%.7f", "2D data"=w637, "file path (dialog if empty)"=w635) -> ()  [unwired: 4 in, 1 out]
                    }
                  }
                }
              }
              n349 = global write "GlobalUI.vi" "SW Initializing"(FALSE ("SW Initializing")) -> ()
            }
          }
        }
        n350 = local write "Save paths"(w576) -> ()
      }
    }
    n351 = Unbundle By Name(w86) -> ("status"=w93:bool)
    n352 = local read "STOP"() -> (w76:bool)
    n353 = Or(x=w93, y=w76) -> (x .or. y?=w92:bool)
    "Numeric" <- w91
  }
